vi "ZMC Execute Get Receive.vi"(0 "handle":u32, 1 "pbifExcuteDown":string, 5 "pbuff":string, 7 "uimax":u32, 9 "puiread":u32, 11 "error in (no error)":errorcluster caption="错误输入（无错误）") -> (3 "pbifExcuteDown out":string, 4 "handle out":u32, 6 "pbuff out":string, 8 "function return":i32, 10 "puiread out":u32, 15 "error out":errorcluster caption="错误输出")   [LabVIEW 2015, in "zauxdll.lvlib"]
doc: "int32 __stdcall ZMC_ExecuteGetReceive(ZMC_HANDLE handle, char * pbuff, uint32 uimax, uint32 *puiread, uint8 *pbifExcuteDown);"
uses:
  zauxdll.lvlib
  zmotion.dll
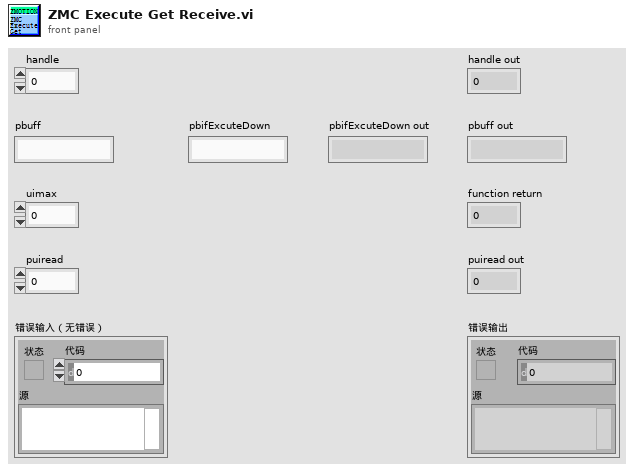
[diagram p1: front panel]
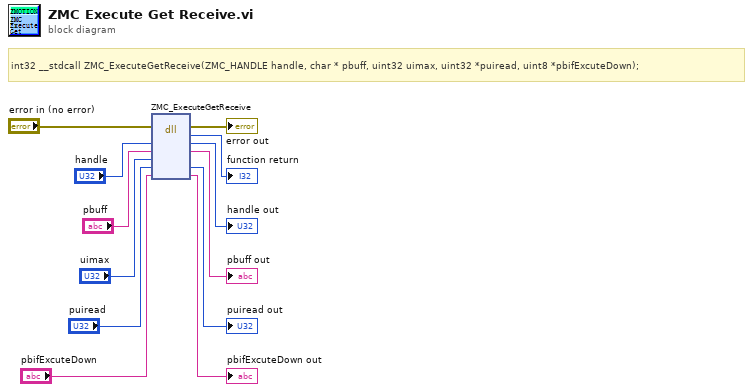
[diagram p0: block diagram]
diagram:
  # "int32 __stdcall ZMC_ExecuteGetReceive(ZMC_HANDLE handle, char * pbuff, uint32 uimax, uint32 *puiread, uint8 *pbifExcuteDown);"
  n1 = dll-call lib="C:/Users/VIC/Desktop/GOGORO_SA/system/LLB/zmotion/zaux/zmotion.*" fn="ZMC_ExecuteGetReceive"(error in="error in (no error)", "handle"="handle", "pbuff"="pbuff", "uimax"="uimax", "puiread"="puiread", "pbifExcuteDown"="pbifExcuteDown") -> (error out=→"error out":errorcluster, →"function return":i32, "handle"=→"handle out":u32, "pbuff"=→"pbuff out":string, "puiread"=→"puiread out":u32, "pbifExcuteDown"=→"pbifExcuteDown out":string)  [unwired: 3 in, 1 out]
